vi "Actor Core.vi"(8 "error in":errorcluster, 11 "CS++DSMonitor in":refnum<class "CS++DSMonitor.lvclass">) -> (0 "error out":errorcluster, 3 "Actor out":refnum<class "Actor.lvclass">)   [LabVIEW 2015, in "CS++DSMonitor.lvlib" / "CS++DSMonitor.lvclass"]
doc: "(<B>Filename</B>: Actor Framework.lvlib:Actor.lvclass:Actor Core.vi)\n\nReceives messages to the actor, reacts to them, and initiates any error handling that may shut the actor down.\n\nDescendant classes may override this VI to append parallel tasks for the actor to complete while it handles messages. Overrides use the Call Parent Method node."
uses:
  CS++DSMonitor.lvclass
  <vilib>/ActorFramework/Actor/Actor.lvclass
  CS++BaseActor/CS++BaseActor.lvclass/CS++BaseActor.ctl
  CS++DSMonitor.lvclass/CS++DSMonitor.ctl
  CS++PVMonitor/CS++PVMonitor.lvclass/CS++PVMonitor.ctl
  Classes/CS++ProcessVariables/ProcessVariable/PV.lvclass
  Classes/CS++ProcessVariables/ProcessVariable/PV.lvclass/PV.ctl
  Classes/CS++ProcessVariables/ProcessVariable/Write PV URL.vi
  Classes/CS++ProcessVariables/ProcessVariable/Write Data.vi
  Classes/CS++ProcessVariables/ProcessVariable/Write Timestamp.vi
  Classes/CS++ProcessVariables/ProcessVariable/Write Error.vi
  Classes/CS++ProcessVariables/ProcessVariable/Write Quality.vi
  Classes/CS++ProcessVariables/ProcessVariable/Write status.vi
  <vilib>/Utility/error.llb/Error Cluster From Error Code.vi
  CS++PVMonitor/CS++PVMonitor.lvclass
  <vilib>/ActorFramework/Message Enqueuer/Message Enqueuer.lvclass
  CS++PVMonitor Messages/CS++PVUpdate Msg/CS++PVUpdate Msg.lvclass
  CS++BaseActor/CS++BaseActor.lvclass
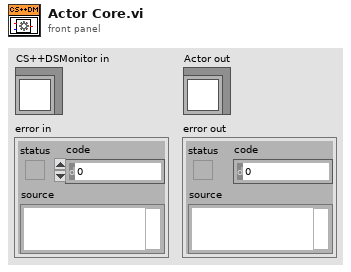
[diagram p1: front panel]
types:
  T1 = cluster{"Stop":refnum<user-event>, "PV Connections":refnum<user-event>}
  T2 = cluster{"Enqueuer":refnum<class "Message Enqueuer.lvclass">, "CS++PVUpdate Msg":refnum<class "CS++PVUpdate Msg.lvclass">}[]
  T3 = cluster{"PV URL":string, "Observers":cluster{"Enqueuer":refnum<class "Message Enqueuer.lvclass">, "CS++PVUpdate Msg":refnum<class "CS++PVUpdate Msg.lvclass">}[]}[]
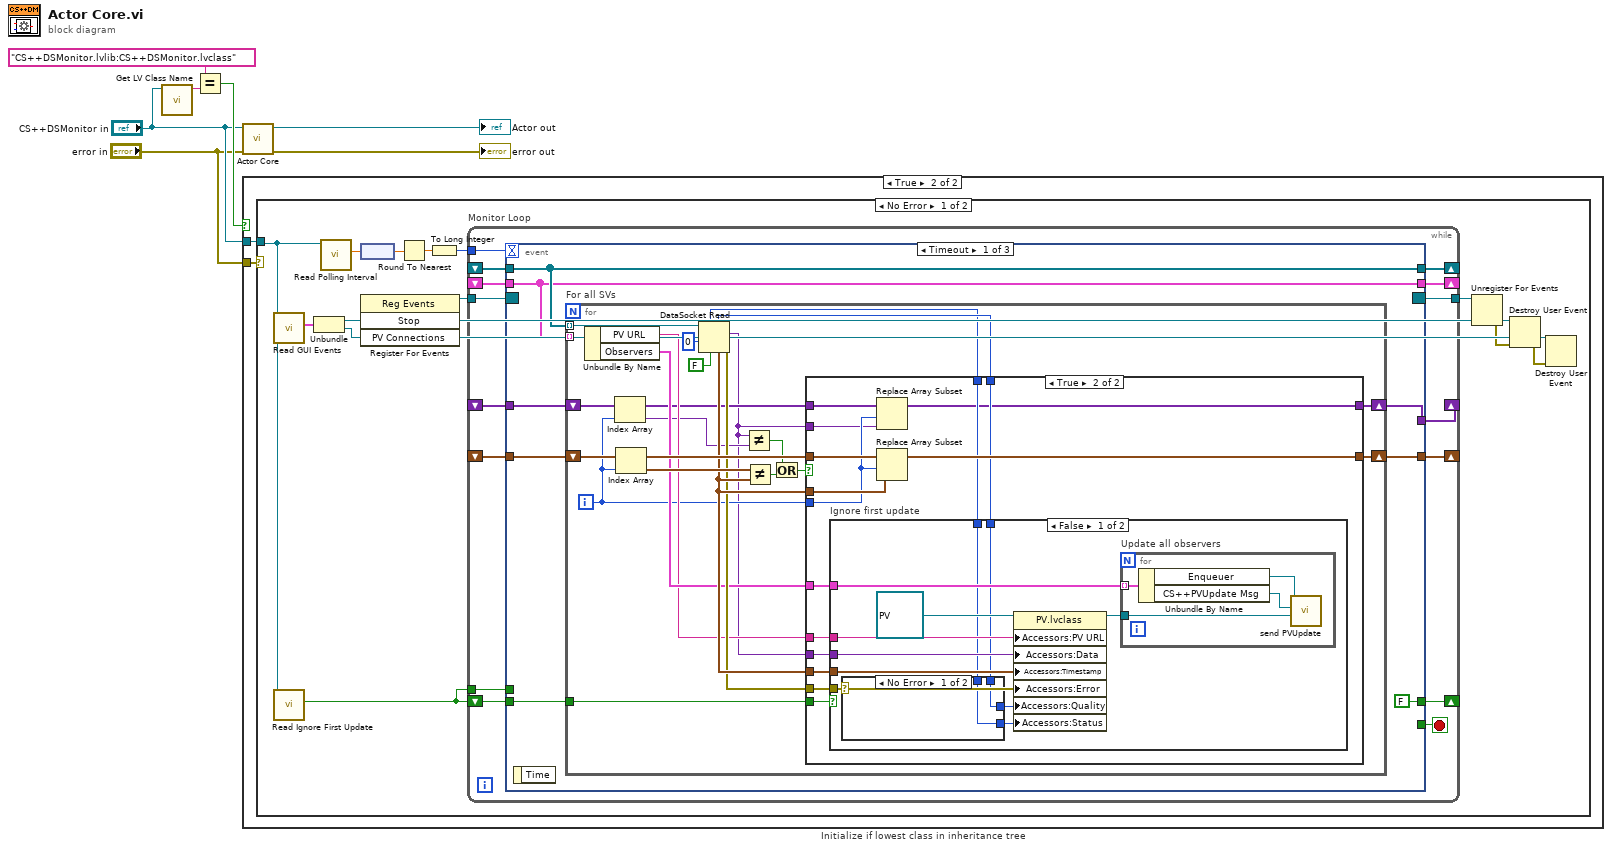
[diagram p0: block diagram]
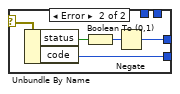
[diagram p4: hidden frame]
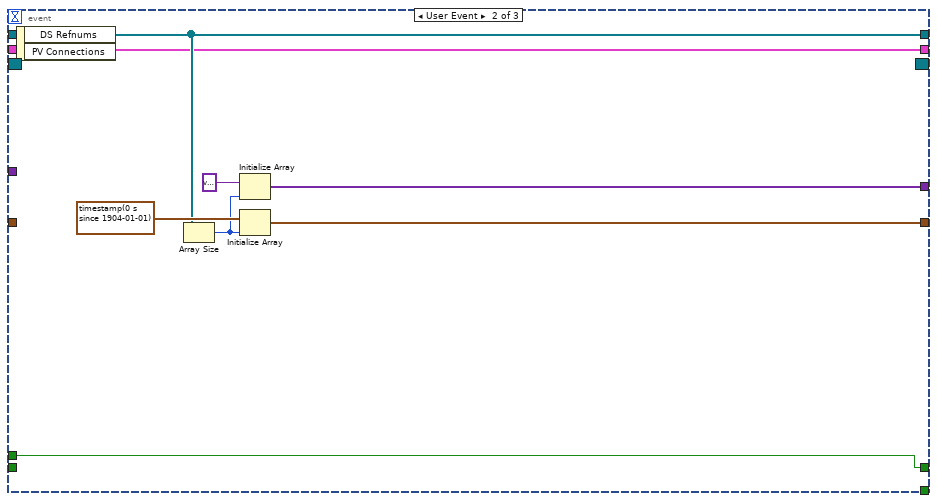
[diagram p6: hidden frame]
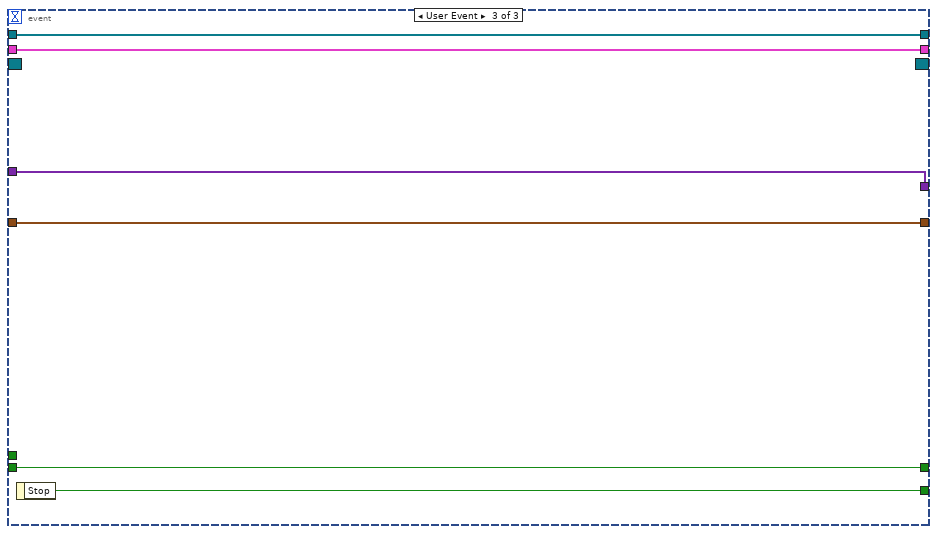
[diagram p7: hidden frame]
diagram:
  n1 = call <vilib>:"Get LV Class Name.vi"("object"="CS++DSMonitor in") -> ("class name"=w4:string)  [unwired: 9 in, 1 out]
  n2 = Equal?(x="CS++DSMonitor.lvlib:CS++DSMonitor.lvclass" ("class name"), y=w4) -> (x = y?=w3:bool)
  n3 = call-parent "Actor Core.vi"("error in"="error in", "CS++BaseActor in"="CS++DSMonitor in") -> ("error out"=→"error out":errorcluster, "Actor out"=→"Actor out":refnum<class "Actor.lvclass">)  [unwired: 8 in]
  n4 = case "Initialize if lowest class in inheritance tree" shown="True" w3 {
    tunnel: "error in" -> [_ w9]
    tunnel: "CS++DSMonitor in" -> [_ w8]
    frame False {
    }
    frame True {
      n5 = case shown="No Error" w9 {
        tunnel: w8 -> [w11 _]
        frame No Error {
          n6 = call "Read GUI Events.vi"("CS++DSMonitor in"=w11) -> ("GUI Events"=w17:T1)  [unwired: 8 in, 2 out]
          n7 = call "Read Ignore First Update.vi"("CS++PVMonitor in"=w11) -> ("Ignore First Update"=w10:bool)  [unwired: 8 in, 2 out]
          n8 = Unbundle(w17) -> ("Stop"=w15:refnum<user-event>, "PV Connections"=w14:refnum<user-event>)
          n9 = call "Read Polling Interval.vi"("CS++BaseActor in"=w11) -> ("Polling Interval"=w20:dbl[unit])  [unwired: 8 in, 2 out]
          n10 = node(w20) -> (w21:dbl)
          n11 = register-events(w15, w14) -> (reference out=w18:refnum<event-registration>)  [unwired: 2 in, 1 out]
          n12 = Round To Nearest(number=w21) -> (nearest integer value=w22:dbl)
          n13 = To Long Integer(number=w22) -> (32bit integer=w19:i32)
          n14 = while "Monitor Loop" {
            tunnel: w18 -> [w37]
            tunnel: w19 -> [w36]
            tunnel: [w34] -> w16
            shift-right: [w32] -> _
            shift-left: _ -> [w33]
            shift-right: [w30] -> _
            shift-left: _ -> [w31]
            shift-right: [w29] -> _
            shift-left: _ -> [w28]
            shift-right: [w27] -> _
            shift-left: _ -> [w26]
            shift-right: [w24] -> _
            shift-left: w10 -> [w25]
            tunnel: w10 -> [w23]
            stop <- w35 stop-if-true
            n15 = event shown="[0] Timeout" {
              selector: w37 -> [_ _ _]
              dyn-events: [_ _ _] -> w34
              timeout: w36 -> [_ _ _]
              tunnel: [_ _ w120] -> w35
              tunnel: w33 -> [w45 _ w119]
              tunnel: [w44 w112 w119] -> w32
              tunnel: w31 -> [w43 _ w118]
              tunnel: [w43 w113 w118] -> w30
              tunnel: [w42 w111 w117] -> w29
              tunnel: w28 -> [w42 _ w117]
              tunnel: [w40 w108 w116] -> w27
              tunnel: w26 -> [w41 _ w116]
              tunnel: w25 -> [w39 _ w115]
              tunnel: [FALSE w107 w115] -> w24
              tunnel: w23 -> [_ w107 _]
              event Timeout {
                n16 = event-data() -> ()  [unwired: 1 in, 1 out]
                n17 = for "For all SVs" {
                  shift-right: [w65] -> w44
                  shift-left: w45 -> [w66]
                  tunnel: w43 -> [w61] mode=indexing
                  tunnel: w42 -> [w60] mode=indexing
                  shift-right: [w52] -> w40
                  shift-left: w41 -> [w51]
                  tunnel: w39 -> [w46]
                  i -> [w50]
                  n18 = Unbundle By Name(w60) -> ("PV URL"=w58:string, "Observers"=w59:T2)
                  n19 = Index Array(array=w51, index=w50) -> (element=w49:variant)
                  n20 = Index Array(array=w66, index=w50) -> (element=w67:timestamp)
                  n21 = DataSocket Read(6:FALSE ("wait for updated value (T)"), 9:0 ("ms timeout (10000)"), 11:w61) -> (0:w62:errorcluster, 2:w48:variant, 4:w63:timestamp, 5:w56:u64, 7:w55:u32)  [unwired: 2 in, 2 out]
                  n22 = Not Equal?(x=w48, y=w49) -> (x != y?=w47:bool)
                  n23 = Not Equal?(x=w67, y=w63) -> (x != y?=w64:bool)
                  n24 = Or(x=w47, y=w64) -> (x .or. y?=w53:bool)
                  n25 = case shown="True" w53 {
                    tunnel: w63 -> [_ w84]
                    tunnel: w66 -> [w69 w83]
                    tunnel: w50 -> [_ w73]
                    tunnel: [w69 w82] -> w65
                    tunnel: w48 -> [_ w79]
                    tunnel: w63 -> [_ w78]
                    tunnel: w62 -> [_ w77]
                    tunnel: w59 -> [_ w81]
                    tunnel: w58 -> [_ w80]
                    tunnel: w56 -> [_ w76]
                    tunnel: w55 -> [_ w75]
                    tunnel: w51 -> [w68 w74]
                    tunnel: [w68 w71] -> w52
                    tunnel: w48 -> [_ w72]
                    tunnel: w46 -> [_ w70]
                    frame False {
                    }
                    frame True {
                      n26 = case "Ignore first update" shown="False" w70 {
                        tunnel: w81 -> [w95 _]
                        tunnel: w80 -> [w92 _]
                        tunnel: w79 -> [w91 _]
                        tunnel: w78 -> [w90 _]
                        tunnel: w77 -> [w89 _]
                        tunnel: w76 -> [w86 _]
                        tunnel: w75 -> [w85 _]
                        frame False {
                          n27 = case shown="No Error" w89 {
                            selector: w89 -> [_ w98]
                            tunnel: [w96 w102] -> w94
                            tunnel: [w97 w101] -> w93
                            tunnel: w86 -> [w97 _]
                            tunnel: w85 -> [w96 _]
                            frame No Error {
                            }
                            frame Error {
                              n28 = Unbundle By Name(w98) -> ("status"=w99:bool, "code"=w102:i32)
                              n29 = Boolean To (0,1)(Boolean=w99) -> (0, 1=w100:i16)
                              n30 = Negate(x=w100) -> (-x=w101:i16)
                            }
                          }
                          n31 = property class="PV.lvclass"(reference=refnum<class "PV.lvclass"> refnum ("PV"), "Accessors:PV URL"=w92, "Accessors:Data"=w91, "Accessors:Timestamp"=w90, "Accessors:Error"=w89, "Accessors:Quality"=w93, "Accessors:Status"=w94) -> (reference out=w87:refnum<class "PV.lvclass">)  [unwired: 1 in, 1 out]
                          n32 = for "Update all observers" {
                            tunnel: w95 -> [w106] mode=indexing
                            tunnel: w87 -> [w103]
                            n33 = Unbundle By Name(w106) -> ("Enqueuer"=w105:refnum<class "Message Enqueuer.lvclass">, "CS++PVUpdate Msg"=w104:refnum<class "CS++PVUpdate Msg.lvclass">)
                            n34 = call "send PVUpdate.vi"("PV"=w103, "CS++PVUpdate Msg in"=w104, "Message Enqueuer in"=w105) -> ()  [unwired: 7 in, 2 out]
                          }
                        }
                        frame True {
                        }
                      }
                      n35 = Replace Array Subset(array=w74, new element=w72, index=w73) -> (w71:variant[])
                      n36 = Replace Array Subset(array=w83, new element=w84, index=w73) -> (w82:timestamp[])
                    }
                  }
                }
              }
              event User Event {
                n37 = event-data() -> ("DS Refnums"=w113:refnum<k13>[], "PV Connections"=w111:T3)  [unwired: 1 in]
                n38 = Array Size(array=w113) -> (size(s)=w110:i32)
                n39 = Initialize Array(variant, w110) -> (w108:variant[])
                n40 = Initialize Array(timestamp(0 s since 1904-01-01) ("timestamp"), w110) -> (w112:timestamp[])
              }
              event User Event {
                n41 = event-data() -> ("Stop"=w120:bool)  [unwired: 1 in]
              }
            }
          }
          n42 = Unregister For Events(event registration refnum=w16) -> (error out=w13:errorcluster)  [unwired: 1 in]
          n43 = Destroy User Event(user event=w15, error in=w13) -> (error out=w12:errorcluster)
          n44 = Destroy User Event(user event=w14, error in=w12) -> ()  [unwired: 1 out]
        }
        frame Error {
        }
      }
    }
  }
